vi "SetClawOpen.vi"(7 "Reinit":bool, 8 "arguments":string[](array[string]), 9 "dt":i32, 10 "SensorInputData":T2, 11 "HMI to Control":T1) -> (2 "SensorInputDataOut":T2, 3 "HMI to ControlOut":T1, 4 "Done":bool=TRUE)   [LabVIEW 2015]
uses:
  Typedefs/ClawStates.ctl
  Typedefs/SensorInputData.ctl
  Typedefs/HMI_to_Control.ctl
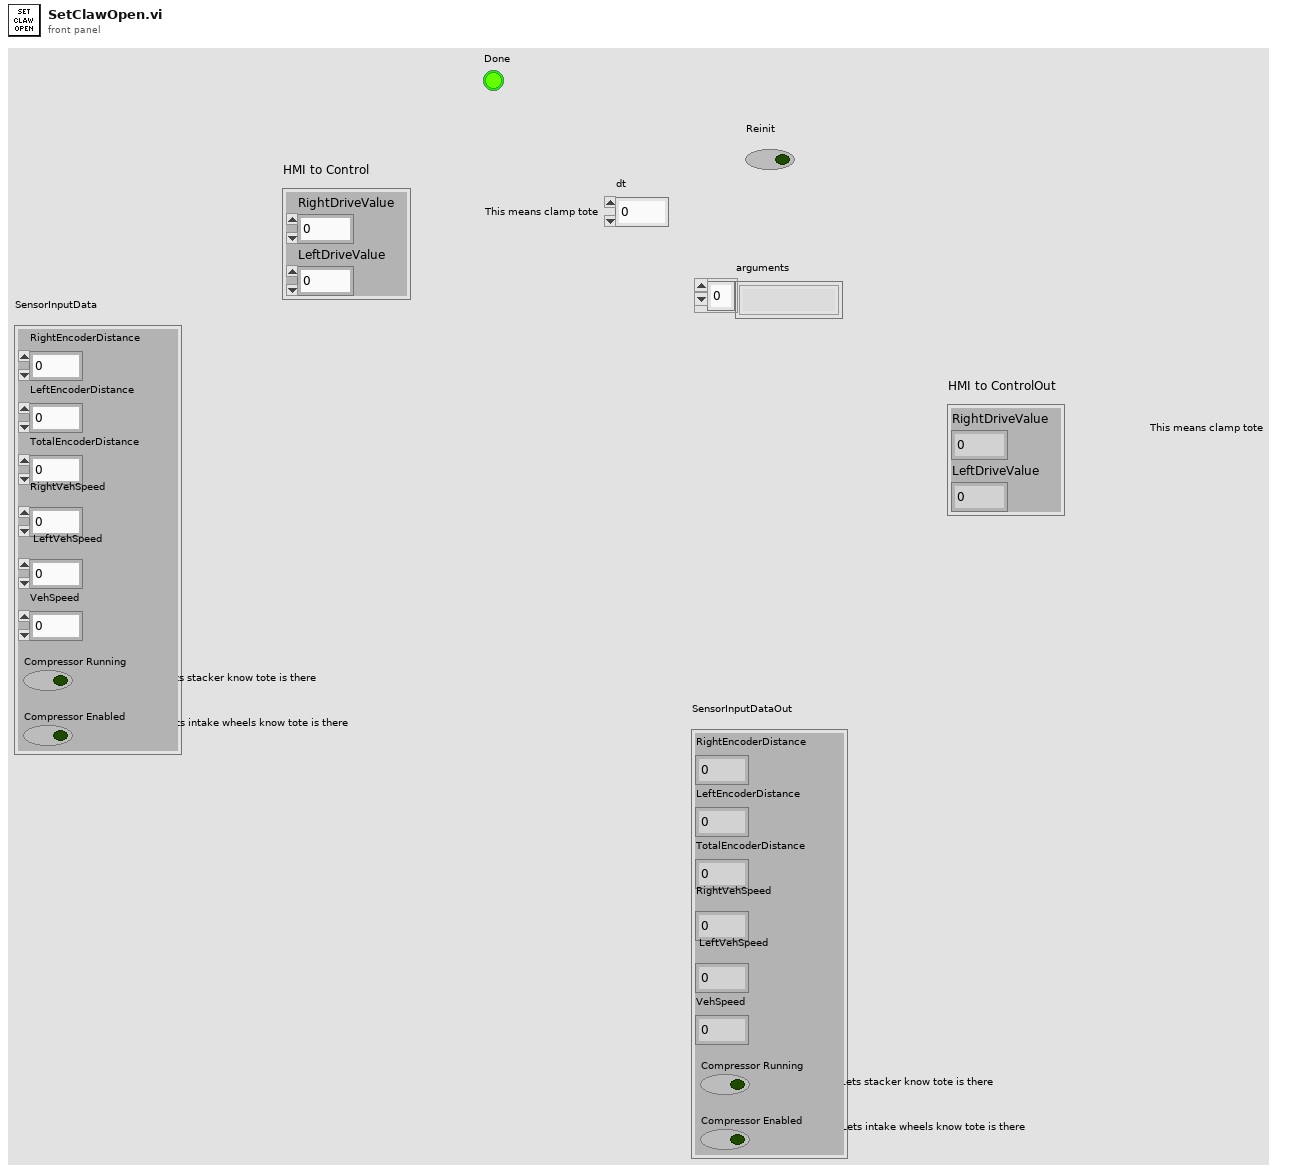
[diagram p1: front panel]
types:
  T1 = typedef "HMI_to_Control.ctl" = cluster{"RightDriveValue":dbl, "LeftDriveValue":dbl}
  T2 = typedef "SensorInputData.ctl" = cluster{"RightEncoderDistance":dbl, "LeftEncoderDistance":dbl, "TotalEncoderDistance":dbl, "RightVehSpeed":dbl, "LeftVehSpeed":dbl, "VehSpeed":dbl, "Compressor Running":bool, "Compressor Enabled":bool}
  T3 = typedef "ClawStates.ctl" = enum16{"Claw Manual ", "Claw Open", "Claw Closed", "Claw Slight Open", "Flip Can"}
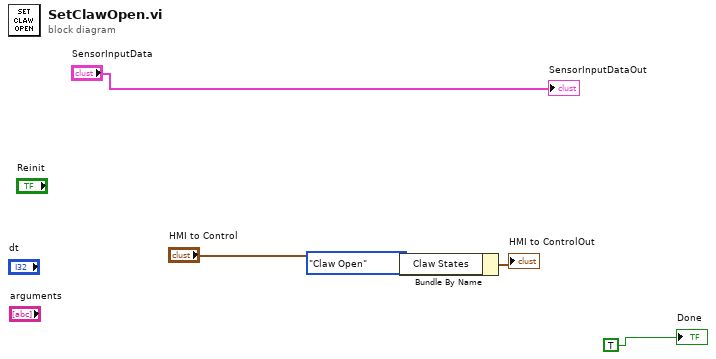
[diagram p0: block diagram]
diagram:
  n1 = Bundle By Name(cluster="HMI to Control", "Claw States"=ClawStates."Claw Open") -> (→"HMI to ControlOut":T1)
  "SensorInputDataOut" <- "SensorInputData"
  "Done" <- TRUE
